vi "Update Card.vi"(8 "error in (no error)":errorcluster, 11 "BME_DG_G05P2_Chnl in":refnum<class "BME_DG_G05P2_Chnl.lvclass">) -> (0 "error out":errorcluster, 3 "BME_DG_G05P2_Chnl out":refnum<class "BME_DG_G05P2_Chnl.lvclass">)   [LabVIEW 2009, in "BME_DG_G05P2_Chnl.lvclass"]
uses:
  BME_DG_G05P2_Chnl.lvclass
  BME_DG_G05P2_Chnl.lvclass/BME_DG_G05P2_Chnl.ctl
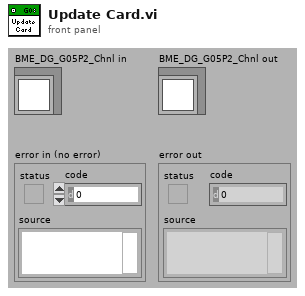
[diagram p1: front panel]
types:
  T1 = typedef "ChnlSettings.ctl" = cluster{" Delay (µs)":dbl, "On? (false)":bool, "PositiveVoltage?(true)":bool, "50OhmTerminated? ":bool, "25OhmOutput?":bool}
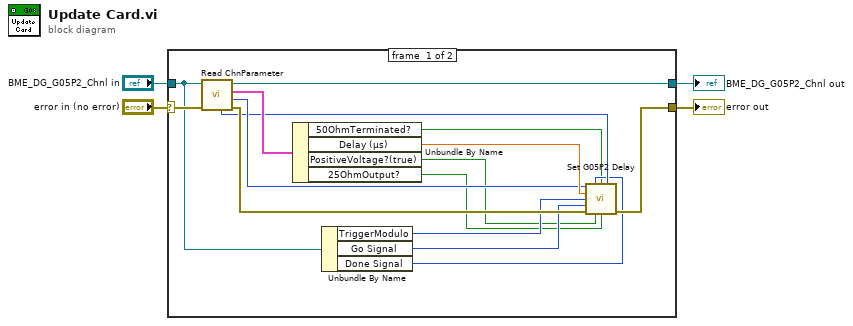
[diagram p0: block diagram]
diagram:
  n1 = case shown="No Error" "error in (no error)" {
    selector: "error in (no error)" -> [w18 w21]
    tunnel: [w16 w21] -> w1
    tunnel: [w14 w20] -> w3
    tunnel: "BME_DG_G05P2_Chnl in" -> [w5 w20]
    frame #0 {
      n2 = call-dynamic "Read ChnParameter.vi"("error in (no error)"=w18, "BME_DG_Chnl in"=w5) -> ("error out"=w17:errorcluster, "Nr"=w12:i32, "ChnParemater"=w19:T1, "BME_DG_Chnl out"=w14:refnum<class "BME_DG_G05P2_Chnl.lvclass">, "DG Nr"=w11:i32)  [unwired: 4 in, 1 out]
      n3 = Unbundle By Name(w19) -> ("50OhmTerminated?"=w8:bool, "Delay (µs)"=w15:dbl, "PositiveVoltage?(true)"=w7:bool, "25OhmOutput?"=w6:bool)
      n4 = Unbundle By Name(w5) -> ("TriggerModulo"=w13:i32, "Go Signal"=w10:u32, "Done Signal"=w9:u32)
      n5 = call "Set G05P2 Delay.vi"("Channel"=w12, "DoneSignal"=w9, "Terminate"=w8, "DG Number"=w11, "Delay (µs)"=w15, "OutputModulo"=w13, "GoSignal"=w10, "error in (no error)"=w17, "Polarity"=w7, "High Drive"=w6) -> ("error out"=w16:errorcluster)  [unwired: 5 in]
    }
    frame #1 {
    }
  }
  "error out" <- w1
  "BME_DG_G05P2_Chnl out" <- w3
